vi "append_element.vi"(1 "append_element":dbl format="%#_13g", 2 "input_double_array.lvclass":refnum<class "double_array.lvclass">) -> (0 "output_double_array.lvclass":refnum<class "double_array.lvclass">)   [LabVIEW 2014, in "double_array.lvclass"]
uses:
  double_array.lvclass
  double_array.lvclass/double_array.ctl
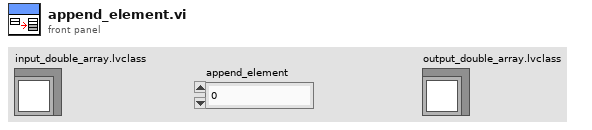
[diagram p1: front panel]
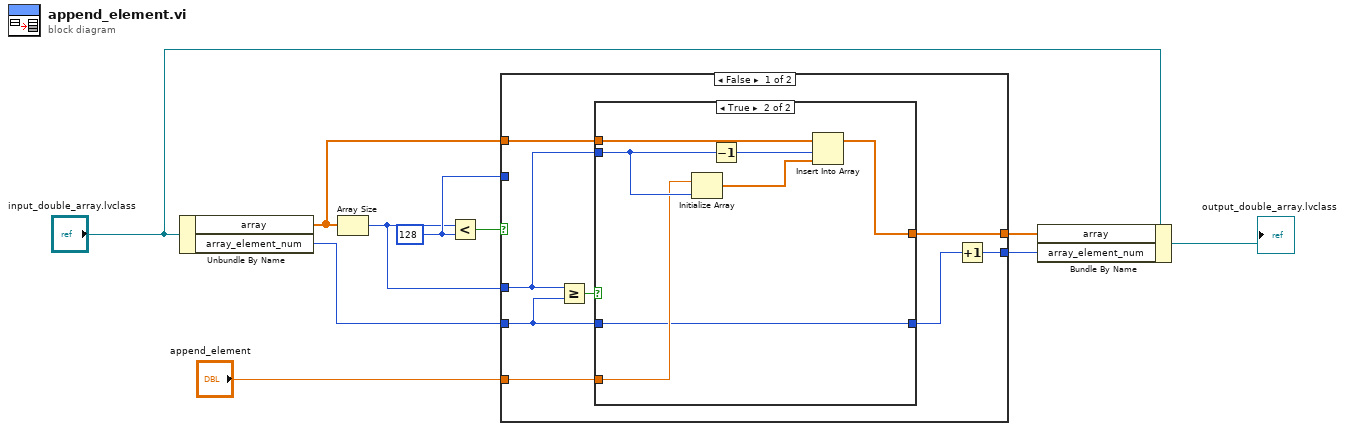
[diagram p0: block diagram]
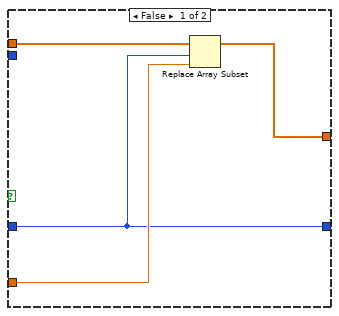
[diagram p2: hidden frame]
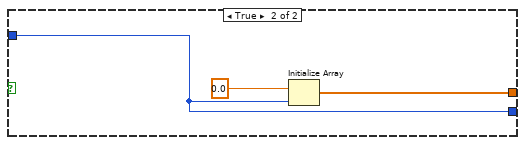
[diagram p3: hidden frame]
diagram:
  w6 = 128 ("y")
  n1 = Unbundle By Name("input_double_array.lvclass") -> ("array"=w2:dbl[], "array_element_num"=w7:u32)
  n2 = Array Size(array=w2) -> (size(s)=w3:i32)
  n3 = Less?(x=w3, y=w6) -> (x < y?=w10:bool)
  n4 = case shown="False" w10 {
    tunnel: w7 -> [w17 _]
    tunnel: w6 -> [_ w30]
    tunnel: [w14 w31] -> w5
    tunnel: [w11 w30] -> w4
    tunnel: w3 -> [w13 _]
    tunnel: w2 -> [w16 _]
    tunnel: "append_element" -> [w15 _]
    frame False {
      n5 = Greater Or Equal?(x=w13, y=w17) -> (x >= y?=w18:bool)
      n6 = case shown="True" w18 {
        tunnel: w17 -> [w19 w23]
        tunnel: w16 -> [w22 w29]
        tunnel: w15 -> [w21 w25]
        tunnel: [w20 w24] -> w14
        tunnel: w13 -> [_ w27]
        tunnel: [w19 w23] -> w12
        frame False {
          n7 = Replace Array Subset(array=w22, new element=w21, index=w19) -> (w20:dbl[])
        }
        frame True {
          n8 = Initialize Array(w25, w27) -> (w26:dbl[])
          n9 = Decrement(x=w27) -> (x-1=w28:i32)
          n10 = Insert Into Array(array=w29, index=w28, new element=w26) -> (w24:dbl[])
        }
      }
      n11 = Increment(x=w12) -> (x+1=w11:u32)
    }
    frame True {
      n12 = Initialize Array(0.0, w30) -> (w31:dbl[])
    }
  }
  n13 = Bundle By Name(cluster="input_double_array.lvclass", "array"=w5, "array_element_num"=w4) -> (→"output_double_array.lvclass":refnum<class "double_array.lvclass">)
